vi "FPGA varible.vi"() -> ()   [LabVIEW 2019]
panel:
  out "FPGA VI Reference":refnum<k20>
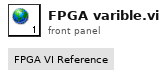
[diagram p1: front panel]
diagram:
